vi "Get DataType Description String.vi"(6 "ignore typedef? (F)":bool, 8 "error in (no error)":errorcluster, 11 "Variant":variant) -> (0 "error out":errorcluster, 3 "String":string)   [LabVIEW 2017]
doc: "This VI shoes the data type of the data stored in Variant input."
uses:
  <vilib>/Utility/Data Type/Type Definitions/Data Type.ctl
  <vilib>/Utility/Data Type/NI_Data Type.lvlib
  _openG/_reuse_openG.lvlib
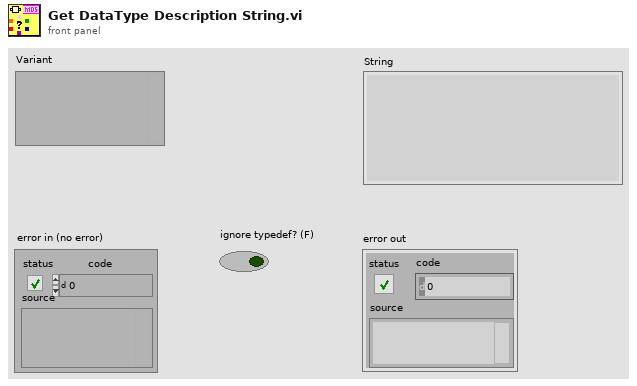
[diagram p1: front panel]
types:
  T1 = typedef "NI_Data Type.lvlib/Data Type.ctl" = enum8{"Invalid Type", "Void", "I8", "I16", "I32", "I64", "U8", "U16", "U32", "U64", "Single Float", "Double Float", "Extended Float", "Single Complex", "Double Complex", "Extended Complex", "Enum U8", "Enum U16", "Enum U32", "Enum U64", "Single Float With Unit", "Double Float With Unit", "Extended Float With Unit", "Single Complex with Unit", "Double Complex with Unit", "Extended Complex with Unit", "Boolean", "String", "Path", "Picture", "Tag", "Array", "Cluster", "Variant", "LV Variant", "Waveform", "Timestamp", "Digital Waveform", "Digital Data", "ExpressData", "Refnum", "External Data", "VI", "Poly VI", "LabVIEW Class Instance", "Fixed Point"}
  T2 = typedef "NI_Data Type.lvlib/Type Definition Info.ctl" = cluster{"Name":string, "Timestamp":u32}
  T3 = typedef "NI_Data Type.lvlib/VI Server Generic Type.ctl" = enum16{"NoType", "\tkLVObjApp=0x1", "\tkLVObjVI", "\tkLVObjGeneric", "\tkLVObjDecoration", "\tkLVObjText", "\tkLVObjControl", "\tkLVObjColorBox", "\tkLVObjBoolean", "\tkLVObjRefNum", "\tkLVObjVariant", "\tkLVObjPath", "\tkLVObjListBox", "\tkLVObjTable", "\tkLVObjArray", "\tkLVObjPicture", "\tkLVObjOleContainer", "\tkLVObjNumeric", "\tkLVObjDigital", "\tkLVObjNamedNumeric", "\tkLVObjColorRamp", "\tkLVObjSlide", "\tkLVObjGraphOrChart", "\tkLVObjWaveformChart", "\tkLVObjWaveformGraph", "\tkLVObjIntensityChart", "\tkLVObjIntensityGraph", "\tkLVObjString", "\tkLVObjIOName", "\tkLVObjComboBox", "\tkLVObjCluster", "\tkLVObjPanel", "\tkLVObjKnob", "\tkLVObjNumWithScale", "\tkLVObjRing", "\tkLVObjEnum", "\tkLVObjGObject", "\tkLVObjPlot", "\tkLVObjCursor", "\tkLVObjNumericText", "\tkLVObjScale", "\tkLVObjColorScale", "\tkLVObjGraphScale", "\tkLVObjColorGraphScale", "\tkLVObjTypedRefNum", "\tkLVObjOldKnobScale", "\tkLVObjMCListbox", "\tkLVObjMeasureData", "\tkLVObjDSCTag", "\tkLVObjDAQName", "\tkLVObjVISAName", "\tkLVObjIVIName", "\tkLVObjSlideScale", "\tkLVObjTabControl", "\tkLVObjPage", "\tkLVObjTabArrayTabControl", "\tkLVObjConPane", "\tkLVObjDAQMXName", "\tkLVObjVIRefNum", "\tkLVObjLVObjRefNum", "\tkLVObjAbsTime", "\tkLVObjDigitalTable", "\tkLVObjUnused", "\tkLVObjUnused2", "\tkLVObjSCLControl", "\tkLVObjSubPanel", "\tkLVObjTreeControl", "\tkLVObjGenClassTagRef", "\tkLVObjGenClassRef", "\tkLVObjRotaryColorScale", "\tkLVObjPlugInDDOControl", "\tkLVObjPlugInDDOClassHolder", "\tkLVObjRadClusControl", "\tkLVObjProject", "\tkLVObjProjectItem", "\tkLVObjPane", "\tkLVObjSplitterBar", "\tkLVObjProjectBuildItem", "\tkLVObjPixmap", "\tkLVObjFacadeVI", "\tkLVObjLibrary", "\tkLVObjVariable", "\tkLVObjPropertyBag", "\tkLVObjXYGraph", "\tkLVObjScene", "\tkLVObjUDClassLibrary", "\tkLVObjUDClassClone", "\tkLVObjMethodVI", "\tkLVObjXCtlLibrary", "\tkLVObjXNodeLibrary", "\tkLVObjScroll", "\tkLVObjLVTarget", "\tkLVObjMixedGraph", "\tkLVObjProvider", "\tkLVObjCopyOperation", "\tkLVObjTargetItem", "\tkLVObjProjectItemType", "\tkLVObjCopyItem", "\tkLVObjCopyConflict", "\tkLVObjCopyExpert", "\tkLVObjSceneGraphDisp", "\tkLVObjPolyVI", "\tkLVObjLVClassDDO", "kLVObjDiagram=0x4000", "\tkLVObjTerminal", "\tkLVObjConstant", "\tkLVObjPathConstant", "\tkLVObjArrayConstant", "\tkLVObjNumericConstant", "\tkLVObjDigitalNumConstant", "\tkLVObjNamedNumericConstant", "\tkLVObjStringConstant", "\tkLVObjClusterConstant", "\tkLVObjFixedConstant", "\tkLVObjControlTerminal", "\tkLVObjFormulaParameter", "\tkLVObjGlobal", "\tkLVObjLocal", "\tkLVObjRightShiftRegister", "\tkLVObjFunction", "\tkLVObjSubVI", "\tkLVObjCallByRef", "\tkLVObjUnitCast", "\tkLVObjStructure", "\tkLVObjLoop", "\tkLVObjMultiframeStructure", "\tkLVObjSequence", "\tkLVObjCaseSelector", "\tkLVObjFormula", "\tkLVObjGrowableFunction", "\tkLVObjBuildClusterArray", "\tkLVObjCompoundArithmetic", "\tkLVObjIndexArray", "\tkLVObjBuildArray", "\tkLVObjNamedBundler", "\tkLVObjCIN", "\tkLVObjCallLibrary", "\tkLVObjObjectFunction", "\tkLVObjProperty", "\tkLVObjInvoke", "\tkLVObjNode", "\tkLVObjBooleanConstant", "\tkLVObjBlockDiagram", "\tkLVObjRingConstant", "\tkLVObjEnumConstant", "\tkLVObjTunnel", "\tkLVObjLoopTunnel", "\tkLVObjSequenceLocal", "\tkLVObjComparison", "\tkLVObjReadWriteFile", "\tkLVObjTypeCast", "\tkLVObjFlattenUnflattenString", "\tkLVObjGPIBReadWrite", "\tkLVObjForLoop", "\tkLVObjWhileLoop", "\tkLVObjScriptNode", "\tkLVObjArrayToCluster", "\tkLVObjFormatScanString", "\tkLVObjWire", "\tkLVObjProbe", "\tkLVObjInnerTerminal", "\tkLVObjLeftShiftRegister", "\tkLVObjPolySubVI", "\tkLVObjPropItem", "\tkLVObjIONameConstant", "\tkLVObjDSCTagConstant", "\tkLVObjDAQNameConstant", "\tkLVObjVISANameConstant", "\tkLVObjIVINameConstant", "\tkLVObjColorBoxConstant", "\tkLVObjControlRefConstant", "\tkLVObjClassSpecifierConstant", "\tkLVObjConfNode", "\tkLVObjMasterWizard", "\tkLVObjStateDiagWizard", "\tkLVObjOuterTerminal", "\tkLVObjDAQMXNameConstant", "\tkLVObjEventStructure", "\tkLVObjFlatSequence", "\tkLVObjGenClassTagRefConstant", "\tkLVObjAbsTimeConstant", "\tkLVObjExternalNode", "\tkLVObjSubWizard", "\tkLVObjScriptNodeParameter", "\tkLVObjStatVIRef", "\tkLVObjComboBoxConstant", "\tkLVObjTimedLoop", "\tkLVObjGenClassDeepCopy", "\tkLVObjGenClassTagFlat", "\tkLVObjGenClassTagFlatRefConstant", "\tkLVObjGenClassFlat", "\tkLVObjSimDiagram", "\tkLVObjCompDiagram", "\tkLVObjSimNode", "\tkLVObjSimDCO", "\tkLVObjBundler", "\tkLVObjUnbundler", "\tkLVObjNamedUnbundler", "\tkLVObjFlatSeqFrame", "\tkLVObjFlatSeqInTun", "\tkLVObjFlatSeqOutTun", "\tkLVObjRefNumConst", "\tkLVObjFlattenString", "\tkLVObjPolySelector", "\tkLVObjXNode", "\tkLVObjSelectorTunnel", "\tkLVObjCommentNode", "\tkLVObjSdfDiagram", "\tkLVObjSDFCompDiagram", "\tkLVObjSdfNode", "\tkLVObjSdfDCO", "\tkLVObjFileDialog", "\tkLVObjTLDCO", "\tkLVObjTimeSeqFrame", "\tkLVObjTimeFlatSequence", "\tkLVObjTimedSequence", "\tkLVObjXDataNode", "\tkLVObjCodeWizard", "\tkLVObjMathScriptNode", "\tkLVObjMathScriptNodeParameter", "\tkLVObjLVClassBDConst"}
  T4 = typedef "NI_Data Type.lvlib/Refnum Type.ctl" = enum16{"NotARefnum", "UnknownRefnum", "Generic", "Datalog", "ByteStream", "Device", "Occurence", "TCPNetConnection", "Auto", "Menu", "Imaq", "Hardware", "DataSocket", "Visa", "IVI", "UDPNetConnection", "Notifier", "Queue", "Irda", "EventReg", "DotNet", "UserEvent", "Callback", "UNUSED_EMPTY_POSITION", "BlueToothNetConnection", "LVObjApp", "LVObjVI", "LVObjUnknown", "GenericClass", "UserDefinedRefnumTag", "DataValue", "RT FIFO", "TDMS File"}
  T5 = typedef "NI_Data Type.lvlib/Tag Type.ctl" = enum16{"kNoTagType", "\tkDSCTagType", "\tkOldDAQTagType", "\tkIVITagType", "\tkVISATagType", "\tkGenClassTagType", "\tkUnusedTagType1", "\tkFPTagType", "\tkMotionTagType", "\tkDAQmxTaskTagType", "\tkDAQmxChannelTagType", "\tkDAQmxScaleTagType", "\tkDAQmxDeviceTagType", "\tkDAQmxTerminalTagType", "\tkDAQmxPhysChanTagType", "\tkDAQmxTriggerTagType", "\tkDAQmxSwitchTagType", "\tkDAQmxSignalTagType", "\tkUnusedTagType2", "\tkCANTaskTagType", "\tkCANInterfaceTagType", "\tkCANChannelTagType", "\tkNumTagTypes"}
  T6 = typedef "LVFixedPointRepRangeTypeDef.ctl" = cluster{"Range Min":dbl, "Range Max":dbl, "Delta":dbl}
  T7 = typedef "LVFixedPointRepBitsTypeDef.ctl" = cluster{"Signed":bool, "Word Length":u32, "Integer Word Length":i32}
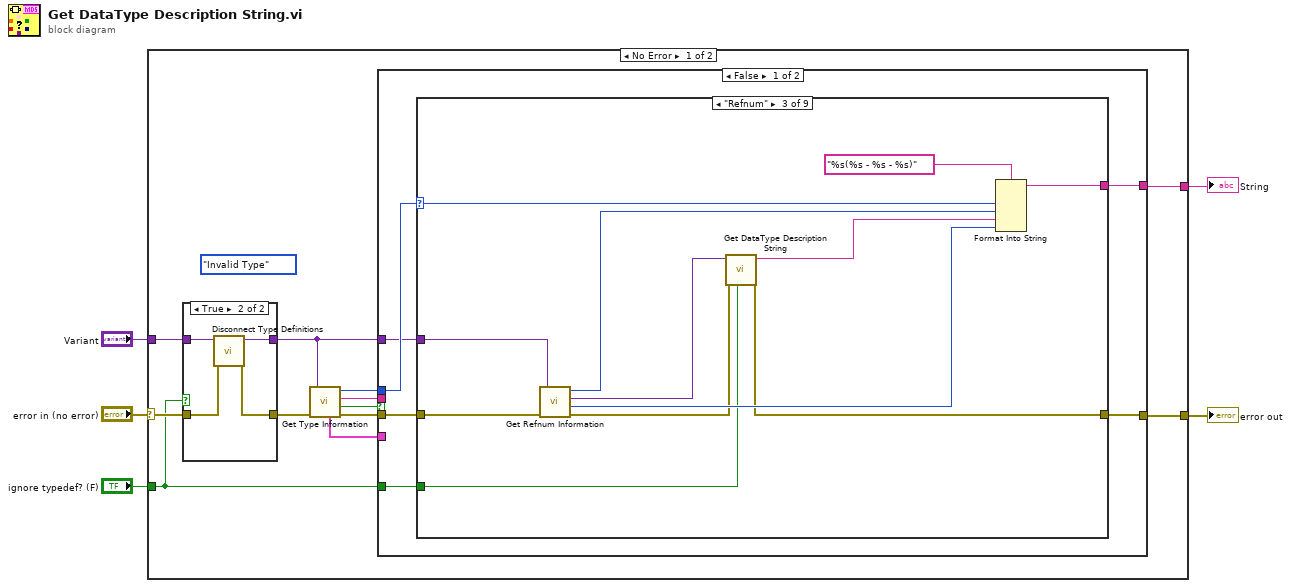
[diagram p0: block diagram]
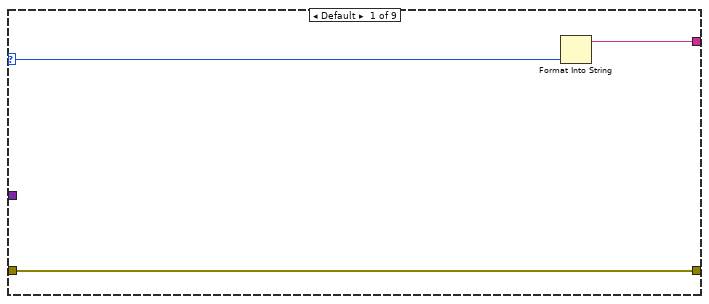
[diagram p3: hidden frame]
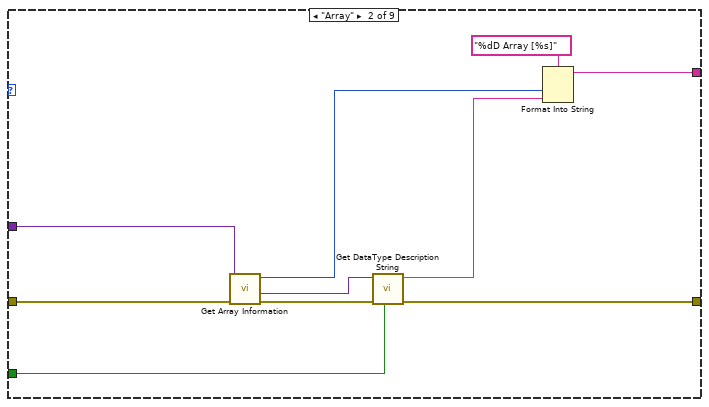
[diagram p4: hidden frame]
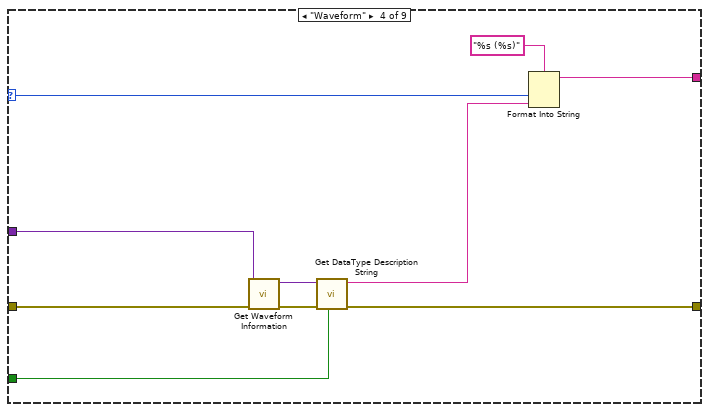
[diagram p5: hidden frame]
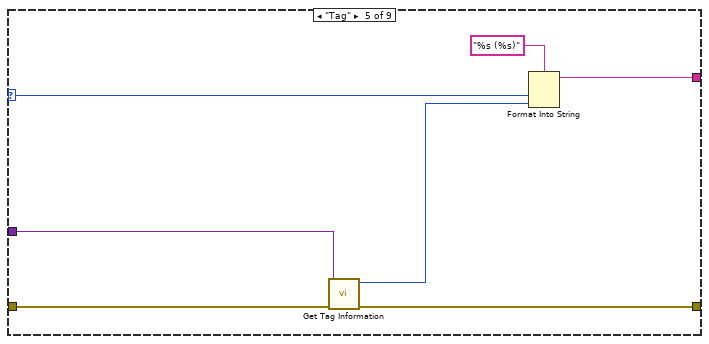
[diagram p6: hidden frame]
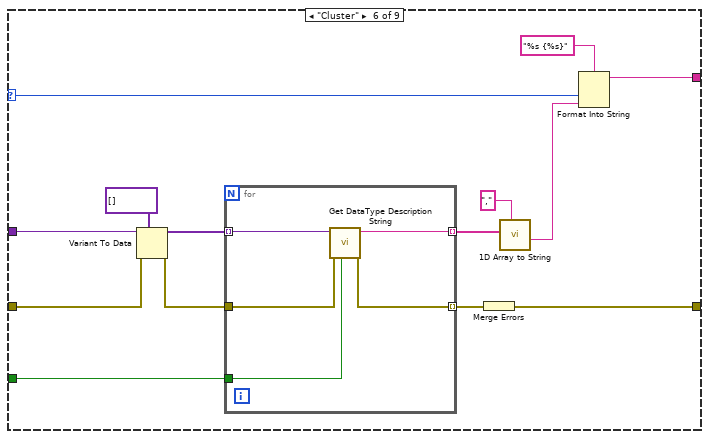
[diagram p7: hidden frame]
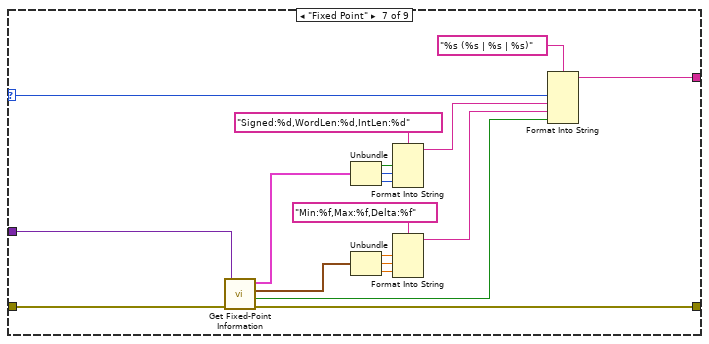
[diagram p8: hidden frame]
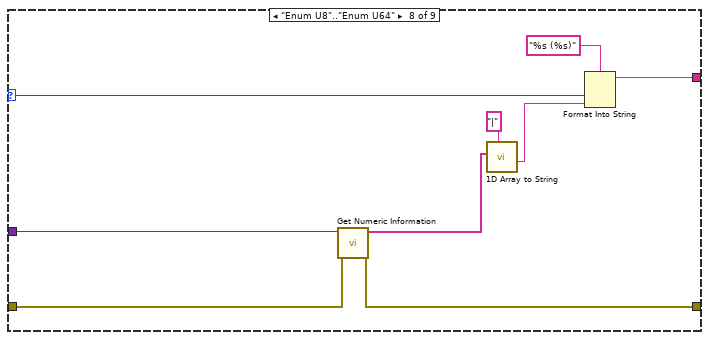
[diagram p9: hidden frame]
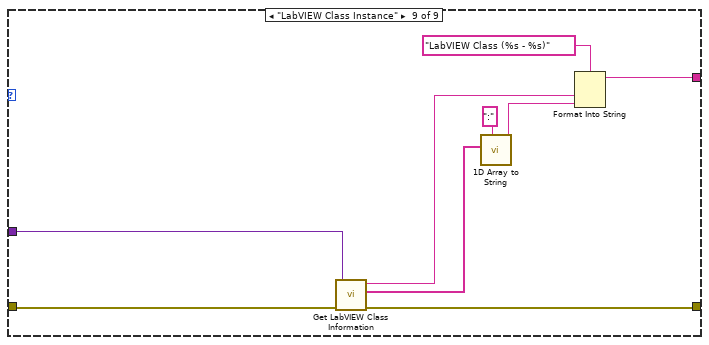
[diagram p10: hidden frame]
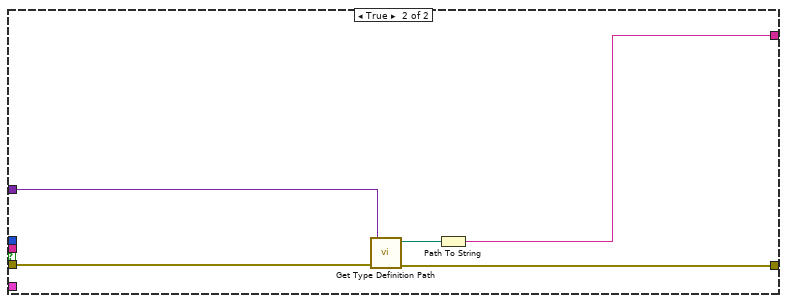
[diagram p11: hidden frame]
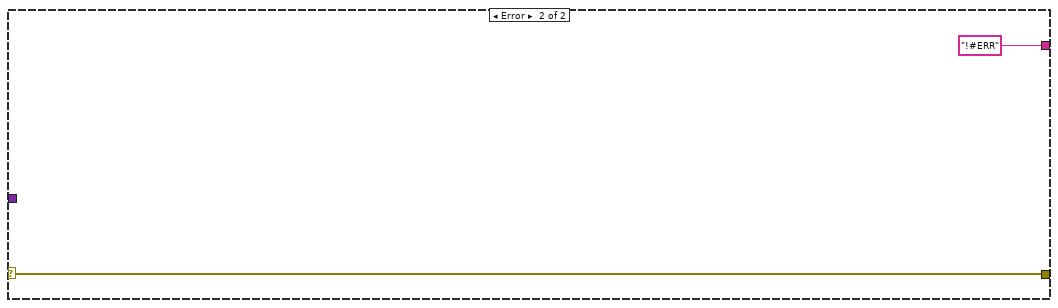
[diagram p12: hidden frame]
diagram:
  n1 = case shown="No Error" "error in (no error)" {
    selector: "error in (no error)" -> [w10 w134]
    tunnel: [w15 w134] -> w5
    tunnel: [w11 "!#ERR"] -> w4
    tunnel: "Variant" -> [w7 _]
    tunnel: "ignore typedef? (F)" -> [w6 _]
    frame No Error {
      (unwired) Data_Type."Invalid Type" ("Type")
      n2 = case shown="True" w6 {
        tunnel: w10 -> [w19 w23]
        tunnel: [w19 w22] -> w9
        tunnel: [w18 w21] -> w8
        tunnel: w7 -> [w18 w20]
        frame False {
        }
        frame True {
          n3 = call <vilib>:"Disconnect Type Definitions.vi"("error in (no error)"=w23, "Variant in"=w20) -> ("error out"=w22:errorcluster, "Variant out"=w21:variant)  [unwired: 8 in]
        }
      }
      n4 = call <vilib>:"Get Type Information.vi"("error in (no error)"=w9, "Variant"=w8) -> ("error out"=w16:errorcluster, "Type Definition"=w17:bool, "Name"=w13:string, "Type"=w14:T1, "Type Definition Info"=w12:T2)  [unwired: 5 in]
      n5 = case shown="False" w17 {
        tunnel: w8 -> [w28 w132]
        tunnel: w16 -> [w27 w131]
        tunnel: [w25 w130] -> w11
        tunnel: [w26 w129] -> w15
        tunnel: w14 -> [w29 _]
        tunnel: w13 -> [_ _]
        tunnel: w12 -> [_ _]
        tunnel: w6 -> [w24 _]
        frame False {
          n6 = case shown="\"Refnum\"" w29 {
            selector: w29 -> [w31 _ w50 w62 w69 w85 w106 w117 _]
            tunnel: w28 -> [_ w42 w53 w63 w70 w73 w108 w113 w126]
            tunnel: w27 -> [w30 w41 w54 w64 w71 w75 w109 w111 w127]
            tunnel: [w30 w34 w43 w55 w66 w80 w107 w110 w125] -> w26
            tunnel: [w32 w38 w51 w61 w68 w84 w105 w114 w122] -> w25
            tunnel: w24 -> [_ w33 w46 w57 _ w79 _ _ _]
            frame Default {
              n7 = Format Into String(w31) -> (resulting string=w32:string)  [unwired: 3 in, 1 out]
            }
            frame "Array" {
              n8 = call <vilib>:"Get Array Information.vi"("error in (no error)"=w41, "Variant"=w42) -> ("error out"=w35:errorcluster, "Array Element Data Type"=w37:variant, "Number of Dimensions"=w39:i32)  [unwired: 6 in, 1 out]
              n9 = call "Get DataType Description String.vi"("ignore typedef? (F)"=w33, "error in (no error)"=w35, "Variant"=w37) -> ("error out"=w34:errorcluster, "String"=w36:string)  [unwired: 7 in]
              n10 = Format Into String(format string="%dD Array [%s]", w39, w36) -> (resulting string=w38:string)  [unwired: 2 in, 1 out]
            }
            frame "Refnum" {
              n11 = call <vilib>:"Get Refnum Information.vi"("error in (no error)"=w54, "Variant"=w53) -> ("error out"=w44:errorcluster, "VI Server Generic Type"=w48:T3, "Strict Type"=w47:variant, "Reference Type"=w52:T4)  [unwired: 6 in]
              n12 = call "Get DataType Description String.vi"("ignore typedef? (F)"=w46, "error in (no error)"=w44, "Variant"=w47) -> ("error out"=w43:errorcluster, "String"=w45:string)  [unwired: 7 in]
              n13 = Format Into String(format string="%s(%s - %s - %s)", w50, w52, w45, w48) -> (resulting string=w51:string)  [unwired: 2 in, 1 out]
            }
            frame "Waveform" {
              n14 = call <vilib>:"Get Waveform Information.vi"("error in (no error)"=w64, "Variant"=w63) -> ("error out"=w58:errorcluster, "Y Array Type"=w59:variant)  [unwired: 8 in]
              n15 = call "Get DataType Description String.vi"("ignore typedef? (F)"=w57, "error in (no error)"=w58, "Variant"=w59) -> ("error out"=w55:errorcluster, "String"=w56:string)  [unwired: 7 in]
              n16 = Format Into String(format string="%s (%s)", w62, w56) -> (resulting string=w61:string)  [unwired: 2 in, 1 out]
            }
            frame "Tag" {
              n17 = call <vilib>:"Get Tag Information.vi"("error in (no error)"=w71, "Variant"=w70) -> ("error out"=w66:errorcluster, "Tag Type"=w65:T5)  [unwired: 8 in]
              n18 = Format Into String(format string="%s (%s)", w69, w65) -> (resulting string=w68:string)  [unwired: 2 in, 1 out]
            }
            frame "Cluster" {
              n19 = Variant To Data(error in=w75, type=variant[] [] ("Array"), Variant=w73) -> (data=w82:variant[], error out=w74:errorcluster)
              n20 = for {
                tunnel: w82 -> [w90] mode=indexing
                tunnel: w74 -> [w89]
                tunnel: [w88] -> w81 mode=indexing
                tunnel: w79 -> [w87]
                tunnel: [w86] -> w78 mode=indexing
                n21 = call "Get DataType Description String.vi"("ignore typedef? (F)"=w87, "error in (no error)"=w89, "Variant"=w90) -> ("error out"=w88:errorcluster, "String"=w86:string)  [unwired: 7 in]
              }
              n22 = Merge Errors(w81) -> (w80:errorcluster)
              n23 = call "1D Array to String.vi"("delimiter (Tab)"="," ("format string"), "Array of Strings"=w78) -> ("delimited string"=w77:string)  [unwired: 9 in]
              n24 = Format Into String(format string="%s {%s}", w85, w77) -> (resulting string=w84:string)  [unwired: 2 in, 1 out]
            }
            frame "Fixed Point" {
              n25 = call <vilib>:"Get Fixed-Point Information.vi"("error in (no error)"=w109, "Variant"=w108) -> ("error out"=w107:errorcluster, "Include Overflow Status?"=w91:bool, "FXP Range"=w103:T6, "FXP Representation"=w94:T7)  [unwired: 6 in]
              n26 = Unbundle(w94) -> ("Signed"=w96:bool, "Word Length"=w95:u32, "Integer Word Length"=w97:i32)
              n27 = Unbundle(w103) -> ("Range Min"=w101:dbl, "Range Max"=w102:dbl, "Delta"=w100:dbl)
              n28 = Format Into String(format string="Signed:%d,WordLen:%d,IntLen:%d", w96, w95, w97) -> (resulting string=w93:string)  [unwired: 2 in, 1 out]
              n29 = Format Into String(format string="Min:%f,Max:%f,Delta:%f", w101, w102, w100) -> (resulting string=w92:string)  [unwired: 2 in, 1 out]
              n30 = Format Into String(format string="%s (%s | %s | %s)", w106, w93, w92, w91) -> (resulting string=w105:string)  [unwired: 2 in, 1 out]
            }
            frame "Enum U8".."Enum U64" {
              n31 = call <vilib>:"Get Numeric Information.vi"("error in (no error)"=w111, "Variant"=w113) -> ("error out"=w110:errorcluster, "Enum Names"=w112:string[])  [unwired: 6 in, 2 out]
              n32 = call "1D Array to String.vi"("delimiter (Tab)"="|", "Array of Strings"=w112) -> ("delimited string"=w115:string)  [unwired: 9 in]
              n33 = Format Into String(format string="%s (%s)", w117, w115) -> (resulting string=w114:string)  [unwired: 2 in, 1 out]
            }
            frame "LabVIEW Class Instance" {
              n34 = call <vilib>:"Get LabVIEW Class Information.vi"("error in (no error)"=w127, "Variant"=w126) -> ("error out"=w125:errorcluster, "Qualified LabVIEW Class Name"=w123:string[], "LabVIEW Class File Name"=w124:string)  [unwired: 7 in]
              n35 = call "1D Array to String.vi"("delimiter (Tab)"=":", "Array of Strings"=w123) -> ("delimited string"=w121:string)  [unwired: 9 in]
              n36 = Format Into String(format string="LabVIEW Class (%s - %s)", w124, w121) -> (resulting string=w122:string)  [unwired: 2 in, 1 out]
            }
          }
        }
        frame True {
          n37 = call <vilib>:"Get Type Definition Path.vi"("error in (no error)"=w131, "Variant"=w132) -> ("error out"=w129:errorcluster, "Type Definition Path"=w128:path)  [unwired: 8 in]
          n38 = Path To String(path=w128) -> (string=w130:string)
        }
      }
    }
    frame Error {
    }
  }
  "String" <- w4
  "error out" <- w5
